vi "Experiment 14.vi"() -> ()   [LabVIEW 2026]
doc: "Experiment 14\nThis experiment is like Experiments 12 and 13 but contains only 2 parallel loops (instead of 10 and 4 as in Exp 12 and Exp 13 respectively)."
uses:
  <vilib>/AdvancedString/1D String Array to Delimited String (string).vi
  <vilib>/Analysis/baseanly.llb/Mean (DBL).vi
  <vilib>/Analysis/NI_AALBase.lvlib
panel:
  out "No. Of Iterations As Block Of Text (easy to copy into Excel)":string
  out "Avg. No. Of Iterations Executed - All Loops":dbl format="%.1f"
  out "No. Of Iterations Executed - Loop 2":i32
  out "Output - Loop 2":dbl[](array[numeric]) format="%.3f"
  out "No. Of Iterations Executed - Loop 1":i32
  out "Output - Loop 1":dbl[](array[numeric]) format="%.3f"
  out "Stop VI?":bool
  # "Experiment 14"
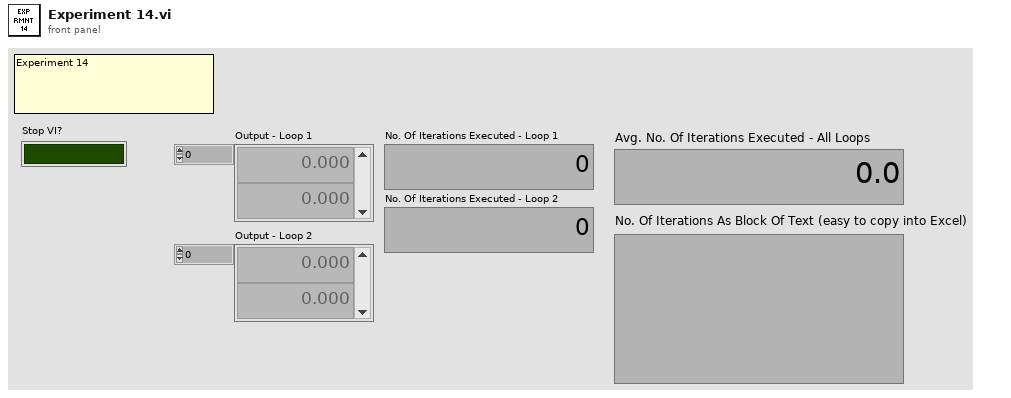
[diagram p1: front panel]
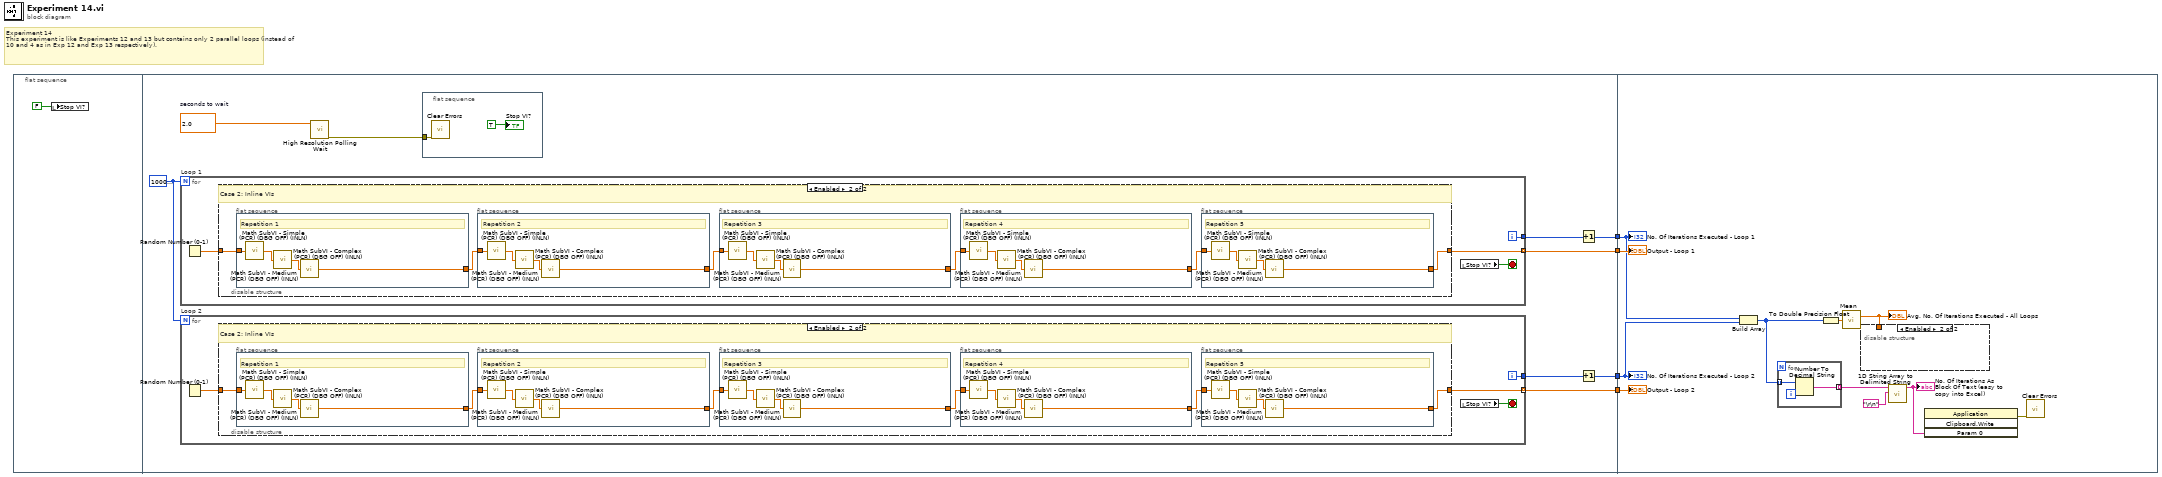
[diagram p0: block diagram]
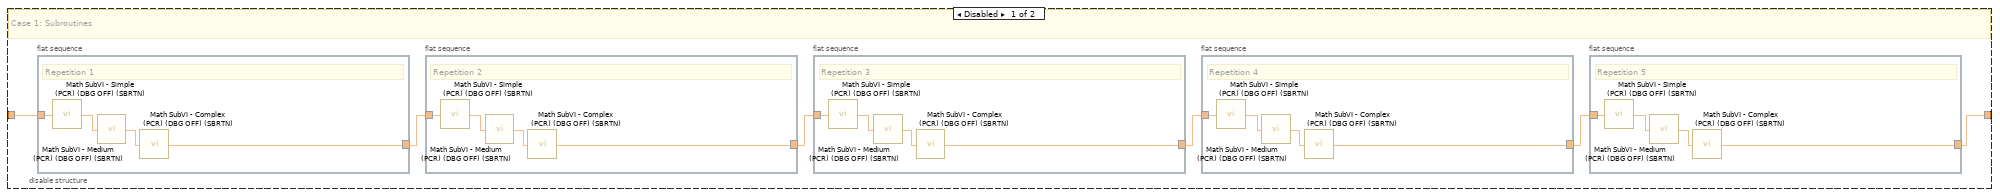
[diagram p2: hidden frame]
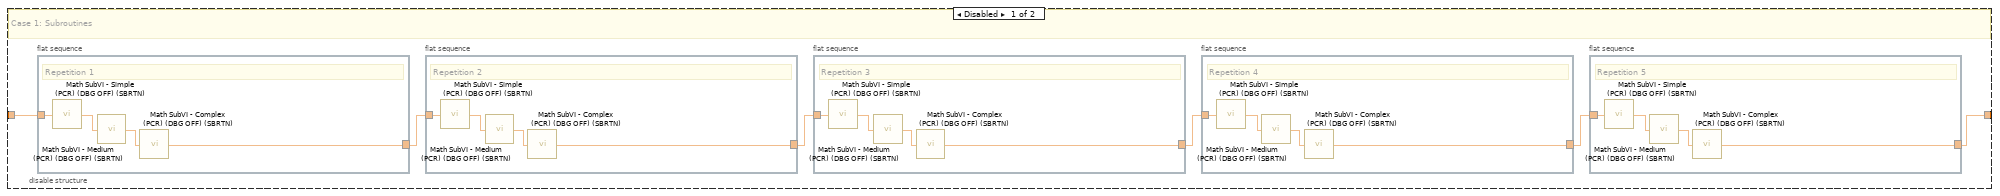
[diagram p3: hidden frame]
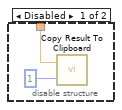
[diagram p4: hidden frame]
diagram:
  # "Experiment 14\nThis experiment is like Experiments 12 and 13 but contains only 2 parallel loops (instead of 10 and 4 as in Exp 12 and Exp 13 respectively)."
  n1 = flat-sequence {
    tunnel: [w12] -> w4
    tunnel: [w10] -> w3
    tunnel: [w9] -> w2
    tunnel: [w8] -> w1
    tunnel: w4 -> [w139]
    tunnel: w3 -> [w137]
    tunnel: w2 -> [w136]
    tunnel: w1 -> [w138]
    frame #0 {
      n2 = local write "Stop VI?"(FALSE) -> ()
    }
    frame #1 {
      w6 = 10000000
      w14 = 2.0  # seconds to wait
      n3 = for "Loop 1" {
        N: w6 -> [_]
        tunnel: [w74] -> w12 mode=indexing
        tunnel: [w75] -> w11
        i -> [w75]
        stop <- w76 stop-if-true
        n4 = Random Number (0-1)() -> (number: 0 to 1=w73:dbl)
        n5 = disable-structure shown="Enabled" {
          disable-tunnel: w73 -> [w82 w108]
          disable-tunnel: [w81 w103] -> w74
          frame Disabled {
            # "Case 1: Subroutines"
            n6 = flat-sequence {
              tunnel: w82 -> [w102]
              tunnel: [w99] -> w77
              frame #0 {
                # "Repetition 1"
                n7 = call "Math SubVI - Simple (PCR) (DBG OFF) (SBRTN).vi"("Input"=w102) -> ("Output"=w100:dbl)
                n8 = call "Math SubVI - Medium (PCR) (DBG OFF) (SBRTN).vi"("Input"=w100) -> ("Output"=w101:dbl)
                n9 = call "Math SubVI - Complex (PCR) (DBG OFF) (SBRTN).vi"("Input"=w101) -> ("Output"=w99:dbl)
              }
            }
            n10 = flat-sequence {
              tunnel: w77 -> [w98]
              tunnel: [w95] -> w80
              frame #0 {
                # "Repetition 2"
                n11 = call "Math SubVI - Simple (PCR) (DBG OFF) (SBRTN).vi"("Input"=w98) -> ("Output"=w96:dbl)
                n12 = call "Math SubVI - Medium (PCR) (DBG OFF) (SBRTN).vi"("Input"=w96) -> ("Output"=w97:dbl)
                n13 = call "Math SubVI - Complex (PCR) (DBG OFF) (SBRTN).vi"("Input"=w97) -> ("Output"=w95:dbl)
              }
            }
            n14 = flat-sequence {
              tunnel: w80 -> [w94]
              tunnel: [w91] -> w79
              frame #0 {
                # "Repetition 3"
                n15 = call "Math SubVI - Simple (PCR) (DBG OFF) (SBRTN).vi"("Input"=w94) -> ("Output"=w92:dbl)
                n16 = call "Math SubVI - Medium (PCR) (DBG OFF) (SBRTN).vi"("Input"=w92) -> ("Output"=w93:dbl)
                n17 = call "Math SubVI - Complex (PCR) (DBG OFF) (SBRTN).vi"("Input"=w93) -> ("Output"=w91:dbl)
              }
            }
            n18 = flat-sequence {
              tunnel: w79 -> [w90]
              tunnel: [w87] -> w78
              frame #0 {
                # "Repetition 4"
                n19 = call "Math SubVI - Simple (PCR) (DBG OFF) (SBRTN).vi"("Input"=w90) -> ("Output"=w88:dbl)
                n20 = call "Math SubVI - Medium (PCR) (DBG OFF) (SBRTN).vi"("Input"=w88) -> ("Output"=w89:dbl)
                n21 = call "Math SubVI - Complex (PCR) (DBG OFF) (SBRTN).vi"("Input"=w89) -> ("Output"=w87:dbl)
              }
            }
            n22 = flat-sequence {
              tunnel: w78 -> [w86]
              tunnel: [w83] -> w81
              frame #0 {
                # "Repetition 5"
                n23 = call "Math SubVI - Simple (PCR) (DBG OFF) (SBRTN).vi"("Input"=w86) -> ("Output"=w84:dbl)
                n24 = call "Math SubVI - Medium (PCR) (DBG OFF) (SBRTN).vi"("Input"=w84) -> ("Output"=w85:dbl)
                n25 = call "Math SubVI - Complex (PCR) (DBG OFF) (SBRTN).vi"("Input"=w85) -> ("Output"=w83:dbl)
              }
            }
          }
          frame Enabled {
            # "Case 2: Inline VIs"
            n26 = flat-sequence {
              tunnel: w108 -> [w128]
              tunnel: [w125] -> w107
              frame #0 {
                # "Repetition 1"
                n27 = call "Math SubVI - Simple (PCR) (DBG OFF) (INLN).vi"("Input"=w128) -> ("Output"=w126:dbl)
                n28 = call "Math SubVI - Medium (PCR) (DBG OFF) (INLN).vi"("Input"=w126) -> ("Output"=w127:dbl)
                n29 = call "Math SubVI - Complex (PCR) (DBG OFF) (INLN).vi"("Input"=w127) -> ("Output"=w125:dbl)
              }
            }
            n30 = flat-sequence {
              tunnel: w107 -> [w124]
              tunnel: [w121] -> w106
              frame #0 {
                # "Repetition 2"
                n31 = call "Math SubVI - Simple (PCR) (DBG OFF) (INLN).vi"("Input"=w124) -> ("Output"=w122:dbl)
                n32 = call "Math SubVI - Medium (PCR) (DBG OFF) (INLN).vi"("Input"=w122) -> ("Output"=w123:dbl)
                n33 = call "Math SubVI - Complex (PCR) (DBG OFF) (INLN).vi"("Input"=w123) -> ("Output"=w121:dbl)
              }
            }
            n34 = flat-sequence {
              tunnel: w106 -> [w120]
              tunnel: [w117] -> w105
              frame #0 {
                # "Repetition 3"
                n35 = call "Math SubVI - Simple (PCR) (DBG OFF) (INLN).vi"("Input"=w120) -> ("Output"=w118:dbl)
                n36 = call "Math SubVI - Medium (PCR) (DBG OFF) (INLN).vi"("Input"=w118) -> ("Output"=w119:dbl)
                n37 = call "Math SubVI - Complex (PCR) (DBG OFF) (INLN).vi"("Input"=w119) -> ("Output"=w117:dbl)
              }
            }
            n38 = flat-sequence {
              tunnel: w105 -> [w116]
              tunnel: [w113] -> w104
              frame #0 {
                # "Repetition 4"
                n39 = call "Math SubVI - Simple (PCR) (DBG OFF) (INLN).vi"("Input"=w116) -> ("Output"=w114:dbl)
                n40 = call "Math SubVI - Medium (PCR) (DBG OFF) (INLN).vi"("Input"=w114) -> ("Output"=w115:dbl)
                n41 = call "Math SubVI - Complex (PCR) (DBG OFF) (INLN).vi"("Input"=w115) -> ("Output"=w113:dbl)
              }
            }
            n42 = flat-sequence {
              tunnel: w104 -> [w112]
              tunnel: [w109] -> w103
              frame #0 {
                # "Repetition 5"
                n43 = call "Math SubVI - Simple (PCR) (DBG OFF) (INLN).vi"("Input"=w112) -> ("Output"=w110:dbl)
                n44 = call "Math SubVI - Medium (PCR) (DBG OFF) (INLN).vi"("Input"=w110) -> ("Output"=w111:dbl)
                n45 = call "Math SubVI - Complex (PCR) (DBG OFF) (INLN).vi"("Input"=w111) -> ("Output"=w109:dbl)
              }
            }
          }
        }
        n46 = local read "Stop VI?"() -> (w76:bool)
      }
      n47 = for "Loop 2" {
        N: w6 -> [_]
        tunnel: [w18] -> w8 mode=indexing
        tunnel: [w19] -> w7
        i -> [w19]
        stop <- w20 stop-if-true
        n48 = Random Number (0-1)() -> (number: 0 to 1=w17:dbl)
        n49 = disable-structure shown="Enabled" {
          disable-tunnel: w17 -> [w26 w52]
          disable-tunnel: [w25 w47] -> w18
          frame Disabled {
            # "Case 1: Subroutines"
            n50 = flat-sequence {
              tunnel: w26 -> [w46]
              tunnel: [w43] -> w21
              frame #0 {
                # "Repetition 1"
                n51 = call "Math SubVI - Simple (PCR) (DBG OFF) (SBRTN).vi"("Input"=w46) -> ("Output"=w44:dbl)
                n52 = call "Math SubVI - Medium (PCR) (DBG OFF) (SBRTN).vi"("Input"=w44) -> ("Output"=w45:dbl)
                n53 = call "Math SubVI - Complex (PCR) (DBG OFF) (SBRTN).vi"("Input"=w45) -> ("Output"=w43:dbl)
              }
            }
            n54 = flat-sequence {
              tunnel: w21 -> [w42]
              tunnel: [w39] -> w24
              frame #0 {
                # "Repetition 2"
                n55 = call "Math SubVI - Simple (PCR) (DBG OFF) (SBRTN).vi"("Input"=w42) -> ("Output"=w40:dbl)
                n56 = call "Math SubVI - Medium (PCR) (DBG OFF) (SBRTN).vi"("Input"=w40) -> ("Output"=w41:dbl)
                n57 = call "Math SubVI - Complex (PCR) (DBG OFF) (SBRTN).vi"("Input"=w41) -> ("Output"=w39:dbl)
              }
            }
            n58 = flat-sequence {
              tunnel: w24 -> [w38]
              tunnel: [w35] -> w23
              frame #0 {
                # "Repetition 3"
                n59 = call "Math SubVI - Simple (PCR) (DBG OFF) (SBRTN).vi"("Input"=w38) -> ("Output"=w36:dbl)
                n60 = call "Math SubVI - Medium (PCR) (DBG OFF) (SBRTN).vi"("Input"=w36) -> ("Output"=w37:dbl)
                n61 = call "Math SubVI - Complex (PCR) (DBG OFF) (SBRTN).vi"("Input"=w37) -> ("Output"=w35:dbl)
              }
            }
            n62 = flat-sequence {
              tunnel: w23 -> [w34]
              tunnel: [w31] -> w22
              frame #0 {
                # "Repetition 4"
                n63 = call "Math SubVI - Simple (PCR) (DBG OFF) (SBRTN).vi"("Input"=w34) -> ("Output"=w32:dbl)
                n64 = call "Math SubVI - Medium (PCR) (DBG OFF) (SBRTN).vi"("Input"=w32) -> ("Output"=w33:dbl)
                n65 = call "Math SubVI - Complex (PCR) (DBG OFF) (SBRTN).vi"("Input"=w33) -> ("Output"=w31:dbl)
              }
            }
            n66 = flat-sequence {
              tunnel: w22 -> [w30]
              tunnel: [w27] -> w25
              frame #0 {
                # "Repetition 5"
                n67 = call "Math SubVI - Simple (PCR) (DBG OFF) (SBRTN).vi"("Input"=w30) -> ("Output"=w28:dbl)
                n68 = call "Math SubVI - Medium (PCR) (DBG OFF) (SBRTN).vi"("Input"=w28) -> ("Output"=w29:dbl)
                n69 = call "Math SubVI - Complex (PCR) (DBG OFF) (SBRTN).vi"("Input"=w29) -> ("Output"=w27:dbl)
              }
            }
          }
          frame Enabled {
            # "Case 2: Inline VIs"
            n70 = flat-sequence {
              tunnel: w52 -> [w72]
              tunnel: [w69] -> w51
              frame #0 {
                # "Repetition 1"
                n71 = call "Math SubVI - Simple (PCR) (DBG OFF) (INLN).vi"("Input"=w72) -> ("Output"=w70:dbl)
                n72 = call "Math SubVI - Medium (PCR) (DBG OFF) (INLN).vi"("Input"=w70) -> ("Output"=w71:dbl)
                n73 = call "Math SubVI - Complex (PCR) (DBG OFF) (INLN).vi"("Input"=w71) -> ("Output"=w69:dbl)
              }
            }
            n74 = flat-sequence {
              tunnel: w51 -> [w68]
              tunnel: [w65] -> w50
              frame #0 {
                # "Repetition 2"
                n75 = call "Math SubVI - Simple (PCR) (DBG OFF) (INLN).vi"("Input"=w68) -> ("Output"=w66:dbl)
                n76 = call "Math SubVI - Medium (PCR) (DBG OFF) (INLN).vi"("Input"=w66) -> ("Output"=w67:dbl)
                n77 = call "Math SubVI - Complex (PCR) (DBG OFF) (INLN).vi"("Input"=w67) -> ("Output"=w65:dbl)
              }
            }
            n78 = flat-sequence {
              tunnel: w50 -> [w64]
              tunnel: [w61] -> w49
              frame #0 {
                # "Repetition 3"
                n79 = call "Math SubVI - Simple (PCR) (DBG OFF) (INLN).vi"("Input"=w64) -> ("Output"=w62:dbl)
                n80 = call "Math SubVI - Medium (PCR) (DBG OFF) (INLN).vi"("Input"=w62) -> ("Output"=w63:dbl)
                n81 = call "Math SubVI - Complex (PCR) (DBG OFF) (INLN).vi"("Input"=w63) -> ("Output"=w61:dbl)
              }
            }
            n82 = flat-sequence {
              tunnel: w49 -> [w60]
              tunnel: [w57] -> w48
              frame #0 {
                # "Repetition 4"
                n83 = call "Math SubVI - Simple (PCR) (DBG OFF) (INLN).vi"("Input"=w60) -> ("Output"=w58:dbl)
                n84 = call "Math SubVI - Medium (PCR) (DBG OFF) (INLN).vi"("Input"=w58) -> ("Output"=w59:dbl)
                n85 = call "Math SubVI - Complex (PCR) (DBG OFF) (INLN).vi"("Input"=w59) -> ("Output"=w57:dbl)
              }
            }
            n86 = flat-sequence {
              tunnel: w48 -> [w56]
              tunnel: [w53] -> w47
              frame #0 {
                # "Repetition 5"
                n87 = call "Math SubVI - Simple (PCR) (DBG OFF) (INLN).vi"("Input"=w56) -> ("Output"=w54:dbl)
                n88 = call "Math SubVI - Medium (PCR) (DBG OFF) (INLN).vi"("Input"=w54) -> ("Output"=w55:dbl)
                n89 = call "Math SubVI - Complex (PCR) (DBG OFF) (INLN).vi"("Input"=w55) -> ("Output"=w53:dbl)
              }
            }
          }
        }
        n90 = local read "Stop VI?"() -> (w20:bool)
      }
      n91 = call <vilib>:"High Resolution Polling Wait.vi"("seconds to wait"=w14) -> ("error out"=w13:errorcluster)  [unwired: 10 in]
      n92 = flat-sequence {
        tunnel: w13 -> [w15]
        frame #0 {
          n93 = call <vilib>:"Clear Errors.vi"("error in (no error)"=w15) -> ()  [unwired: 5 in, 2 out]
          "Stop VI?" <- TRUE
        }
      }
      n94 = Increment(x=w11) -> (x+1=w10:i32)
      n95 = Increment(x=w7) -> (x+1=w9:i32)
    }
    frame #2 {
      n96 = Build Array(w137, w136) -> (w133:i32[])
      n97 = for {
        tunnel: w133 -> [w143] mode=indexing
        tunnel: [w142] -> w132 mode=indexing
        n98 = Number To Decimal String(number=w143) -> (decimal integer string=w142:string)  [unwired: 1 in]
      }
      n99 = To Double Precision Float(number=w133) -> (double precision float=w134:dbl[])
      n100 = call-poly <vilib>:"Mean.vi"("X"=w134) -> ("mean"=w135:dbl)  [unwired: 1 out]
      "Avg. No. Of Iterations Executed - All Loops" <- w135
      n101 = disable-structure shown="Enabled" {
        disable-tunnel: w135 -> [w141 _]
        frame Disabled {
          n102 = call "Copy Result To Clipboard.vi"("No. Of Decimal Places (6)"=u32 1, "Input"=w141) -> ()
        }
        frame Enabled {
        }
      }
      n103 = call-poly <vilib>:"1D String Array to Delimited String.vi"("delimiter"="\r\n", "string array"=w132) -> ("delimited string"=w129:string)  [unwired: 9 in]
      "No. Of Iterations As Block Of Text (easy to copy into Excel)" <- w129
      n104 = invoke class="Application" method="Clipboard.Write"("Param 0"=w129) -> (error out=w130:errorcluster)  [unwired: 3 in, 3 out]
      n105 = call <vilib>:"Clear Errors.vi"("error in (no error)"=w130) -> ()  [unwired: 5 in, 2 out]
      "No. Of Iterations Executed - Loop 1" <- w137
      "Output - Loop 1" <- w139
      "No. Of Iterations Executed - Loop 2" <- w136
      "Output - Loop 2" <- w138
    }
  }
